vi "B29xx_read_ohms(not4user).vi"(4 "Resistance NPLC (0.1)":dbl=0.1, 5 "Resistance Auto Range (T: Enable)":bool=TRUE, 6 "Resistance Range Upper Limit (2E+8 Ohm)":dbl=200000000.0 format="%#_6p", 7 "Enable Remote Sensing (4-wire)":bool=TRUE, 8 "error in (no error)":errorcluster, 9 "Resistance Range (2 Ohm)":dbl=2.0, 10 "Resistance Range Lower Limit (2 Ohm)":dbl=2.0 format="%#_6p", 11 "VISA Refnum in":refnum<visa-resource-name>) -> (0 "error out":errorcluster, 3 "Measurement Result":dbl format="%#_6e")   [LabVIEW 2017]
uses:
  <instrlib>/Agilent B2900 Series/Public/Configure/Measurement/Configure Measurement (Resistance).vi
  <instrlib>/Agilent B2900 Series/Agilent B2900 Series.lvlib
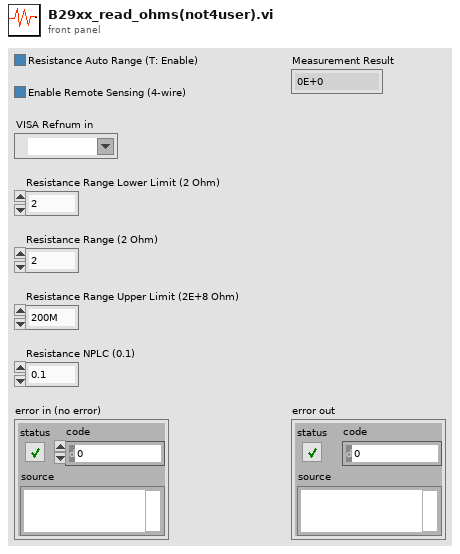
[diagram p1: front panel]
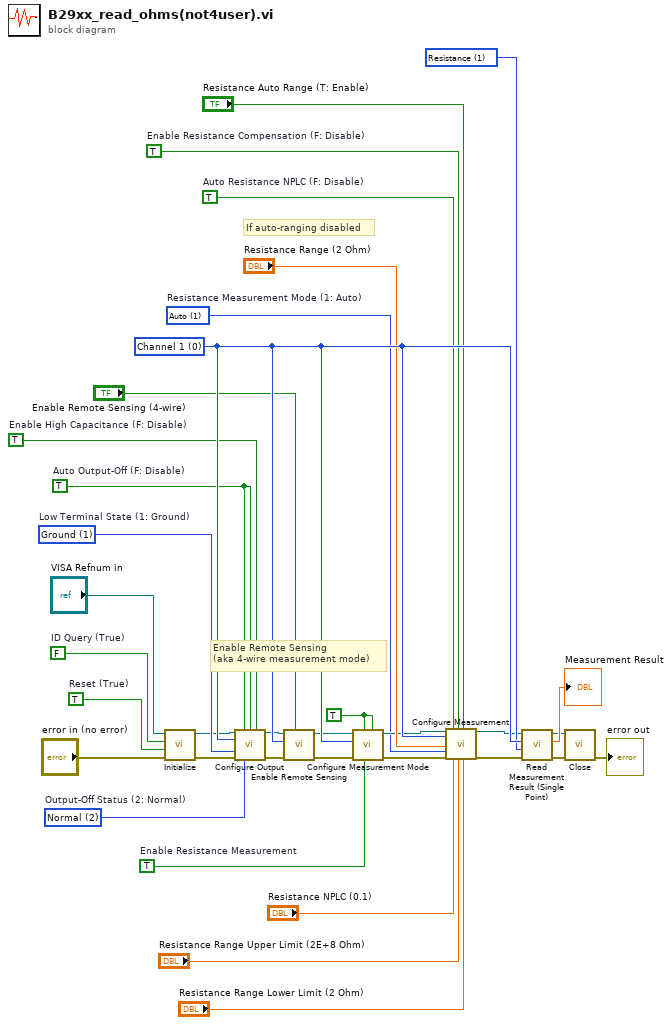
[diagram p0: block diagram]
diagram:
  w31 = 1 items=["Current", "Resistance", "Source Output Setting", "Status", "Time", "Voltage"] ("Data Mode (5: Voltage)")
  w20 = TRUE ("Enable Voltage Measurement (T: Enable)")
  w19 = TRUE  # Enable Resistance Measurement
  w16 = TRUE  # Enable Resistance Compensation (F: Disable)
  w15 = TRUE  # Auto Resistance NPLC (F: Disable)
  w14 = TRUE  # Enable High Capacitance (F: Disable)
  w13 = 1 items=["Manual", "Auto"]  # Resistance Measurement Mode (1: Auto)
  w12 = 2 items=["Zero", "HIZ", "Normal"]  # Output-Off Status (2: Normal)
  w11 = 1 items=["Float", "Ground"]  # Low Terminal State (1: Ground)
  w10 = TRUE  # Auto Output-Off (F: Disable)
  w32 = 0 items=["Channel 1", "Channel 2"] ("Channel (0: Channel 1)")
  w7 = FALSE  # ID Query (True)
  w6 = TRUE  # Reset (True)
  # "If auto-ranging disabled"
  # "Enable Remote Sensing\n(aka 4-wire measurement mode)"
  n1 = call <instrlib>:"Initialize.vi"("error in (no error)"="error in (no error)", "Reset (True)"=w6, "ID Query (True)"=w7, "VISA resource name"="VISA Refnum in") -> ("error out"=w8:errorcluster, "VISA resource name out"=w9:refnum<visa-resource-name>)  [unwired: 6 in]
  n2 = call <instrlib>:"Configure Output.vi"("VISA resource name"=w9, "Auto Output-Off (F: Disable)"=w10, "Auto Output-On (T: Enable)"=w10, "Enable High Capacitance (F: Disable)"=w14, "Channel (0: Channel 1)"=w32, "Low Terminal State (1: Ground)"=w11, "error in (no error)"=w8, "Output-Off Status (2: Normal)"=w12) -> ("VISA resource name out"=w3:refnum<visa-resource-name>, "error out"=w2:errorcluster)  [unwired: 6 in]
  n3 = call <instrlib>:"Enable Remote Sensing.vi"("Enable Remote Sensing (F: Disable)"="Enable Remote Sensing (4-wire)", "error in (no error)"=w2, "Channel (0: Channel 1)"=w32, "VISA resource name"=w3) -> ("error out"=w29:errorcluster, "VISA resource name out"=w30:refnum<visa-resource-name>)  [unwired: 6 in]
  n4 = call <instrlib>:"Configure Measurement Mode.vi"("Enable Current Measurement (T: Enable)"=w20, "Enable Resistance Measurement (F: Disable)"=w19, "Enable Voltage Measurement (T: Enable)"=w20, "error in (no error)"=w29, "Channel (0: Channel 1)"=w32, "VISA resource name"=w30) -> ("error out"=w21:errorcluster, "VISA resource name out"=w22:refnum<visa-resource-name>)  [unwired: 4 in]
  n5 = call-poly <instrlib>:"Configure Measurement.vi"("VISA resource name"=w22, "Channel (0: Channel 1)"=w32, "Resistance Range (2 Ohm)"="Resistance Range (2 Ohm)", "Resistance Measurement Mode (1: Auto)"=w13, "error in (no error)"=w21, "Auto Resistance NPLC (F: Disable)"=w15, "Resistance NPLC (0.1)"="Resistance NPLC (0.1)", "Enable Resistance Compensation (F: Disable)"=w16, "Resistance Range Upper Limit (2E+8 Ohm)"="Resistance Range Upper Limit (2E+8 Ohm)", "Resistance Auto Range (T: Enable)"="Resistance Auto Range (T: Enable)", "Resistance Range Lower Limit (2 Ohm)"="Resistance Range Lower Limit (2 Ohm)") -> ("VISA resource name out"=w24:refnum<visa-resource-name>, "error out"=w23:errorcluster)  [unwired: 7 in]
  n6 = call <instrlib>:"Read Measurement Result (Single Point).vi"("error in (no error)"=w23, "Data Mode (5: Voltage)"=w31, "Channel (0: Channel 1)"=w32, "VISA resource name"=w24) -> ("error out"=w34:errorcluster, "Measurement Result"=→"Measurement Result":dbl, "VISA resource name out"=w33:refnum<visa-resource-name>)  [unwired: 5 in]
  n7 = call <instrlib>:"Close.vi"("error in (no error)"=w34, "VISA resource name"=w33) -> ("error out"=→"error out":errorcluster)  [unwired: 9 in]
